vi "Get Computer Resources.vi"(8 "error in (no error)":errorcluster) -> (0 "error out":errorcluster, 3 "Computer Resources":T1)   [LabVIEW 2020]
doc: "This VI collects via the system data API the available computing resources."
uses:
  Type Definitions/Computer Resources.ctl
  <resource>/objmgr/nicontrollersysapi.rc
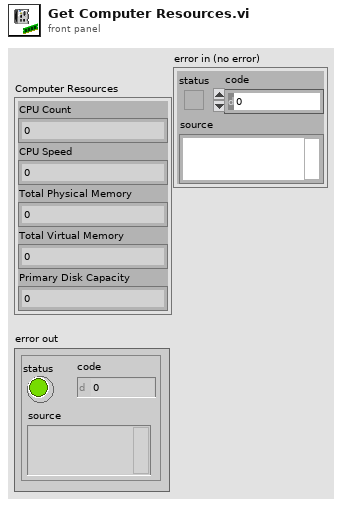
[diagram p1: front panel]
types:
  T1 = typedef "Computer Resources.ctl" = cluster{"CPU Count":i32, "CPU Speed":u32, "Total Physical Memory":dbl, "Total Virtual Memory":dbl, "Primary Disk Capacity":dbl}
  T2 = typedef "System Resources.ctl" = cluster{"System Session":refnum<k21>, "System Resource":refnum<k20>, "FPGA VI Reference":refnum<k20>}
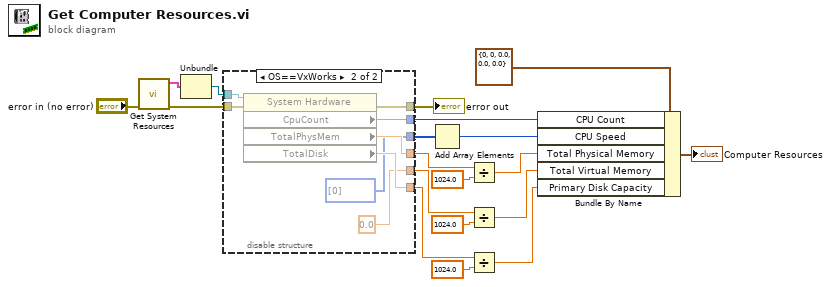
[diagram p0: block diagram]
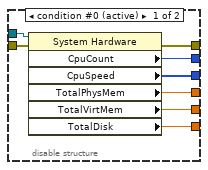
[diagram p2: hidden frame]
diagram:
  n1 = call "Get System Resources.vi"("error in (no error)"="error in (no error)") -> ("error out"=w11:errorcluster, "System Resources"=w14:T2)  [unwired: 9 in]
  n2 = Unbundle(w14) -> ("System Resource"=w13:refnum<k20>)  [unwired: 2 out]
  n3 = disable-structure shown="OS==VxWorks" {
    disable-tunnel: [w27 w35] -> w17
    disable-tunnel: [w26 u32[] [0] ("CpuSpeed")] -> w15
    disable-tunnel: w13 -> [w25 w34]
    disable-tunnel: w11 -> [w24 w33]
    disable-tunnel: [w23 w32] -> w10
    disable-tunnel: [w22 w31] -> w8
    disable-tunnel: [w21 0.0 ("TotalVirtMem")] -> w5
    disable-tunnel: [w20 w30] -> w2
    frame condition #0 (active) {
      n4 = property class="System Hardware"(reference=w25, error in=w24) -> (error out=w23:errorcluster, "CpuCount"=w27:i32, "CpuSpeed"=w26:u32[], "TotalPhysMem"=w20:dbl, "TotalVirtMem"=w21:dbl, "TotalDisk"=w22:dbl)  [unwired: 1 out]
    }
    frame condition #1 {
      n5 = property class="System Hardware"(reference=w34, error in=w33) -> (error out=w32:errorcluster, "CpuCount"=w35:i32, "TotalPhysMem"=w30:dbl, "TotalDisk"=w31:dbl)  [unwired: 1 out]
    }
  }
  "error out" <- w10
  n6 = Add Array Elements(numeric array=w15) -> (sum=w18:u32)
  n7 = Divide(x=w2, y=1024.0) -> (x/y=w1:dbl)
  n8 = Divide(x=w5, y=1024.0) -> (x/y=w4:dbl)
  n9 = Divide(x=w8, y=1024.0) -> (x/y=w7:dbl)
  n10 = Bundle By Name(cluster=T1 {"CPU Count"=0, "CPU Speed"=0, "Total Physical Memory"=0.0, "Total Virtual Memory"=0.0, "Primary Disk Capacity"=0.0}, "CPU Count"=w17, "CPU Speed"=w18, "Total Physical Memory"=w1, "Total Virtual Memory"=w4, "Primary Disk Capacity"=w7) -> (→"Computer Resources":T1)
